vi "CAN_Init - EU.vi"(0 "设备类型":u32(ring)=4 items=["PCI5121"=1, "PCI9810"=2, "USBCAN1"=3, "USBCAN2"=4, "PCI9820"=5, "CAN232"=6, "PCI5110"=7, "CANLite(mini)"=8, "ISA9620"=9, "ISA5420"=10, "PC104CAN"=11, "CANET"=17, "DNP9810"=13, "USBCAN-E-U"=20, "USBCAN-2E-U"=21], 1 "设备索引":u32(ring) items=["0", "1", "2", "3", "4", "5", "6", "7", "8", "9", "10", "11", "12", "13", "14", "15", ""], 2 "波特率":T2(ring)=enum."250Kbps", 3 "CAN路数":u32(ring) items=["0", "1"], 4 "操作类型":enum16{"初始化CAN", "关闭CAN"}(ring), 5 "error in (no error)":errorcluster caption="错误输入（无错误）", 6 "滤波方式":u8(ring)=1 items=["Dual Filter", "Single Filter"], 7 "Accept Code":u32 format="%08x", 8 "IP":string, 9 "port":u32, 10 "工作方式":u8(ring) items=["Normal", "Listen Only"], 11 "Mask Code":u32=4294967295 format="%08x", 12 "PC端-协议类型":enum16{"TCP服务器Server", "TCP客户端Client"}(ring)) -> (14 "CAN 操作结果":bool=TRUE, 19 "error out":errorcluster caption="错误输出")   [LabVIEW 2013]
uses:
  data/ControlCAN.dll
panel:
  in  "VCI_INIT_CONFIG":T1={"AccCode"=0, "AccMask"=4294967295, "Reserved"=0, "Filter"=0, "Timing0"=191, "Timing1"=255, "Mode"=0}
  in  "DeviceType 5":u16(ring)=1 items=["PCI5121"=1, "PCI9810"=2, "USBCAN1"=3, "USBCAN2"=4, "PCI9820"=5, "CAN232"=6, "PCI5110"=7, "CANLite(mini)"=8, "ISA9620"=9, "ISA5420"=10, "PC104CAN"=11, "CANETE"=12, "DNP9810"=13]
  in  "CAN Channel 3":u16(ring) items=["0", "1"]
  in  "DeviceType 4":u16(ring)=1 items=["PCI5121"=1, "PCI9810"=2, "USBCAN1"=3, "USBCAN2"=4, "PCI9820"=5, "CAN232"=6, "PCI5110"=7, "CANLite(mini)"=8, "ISA9620"=9, "ISA5420"=10, "PC104CAN"=11, "CANETE"=12, "DNP9810"=13]
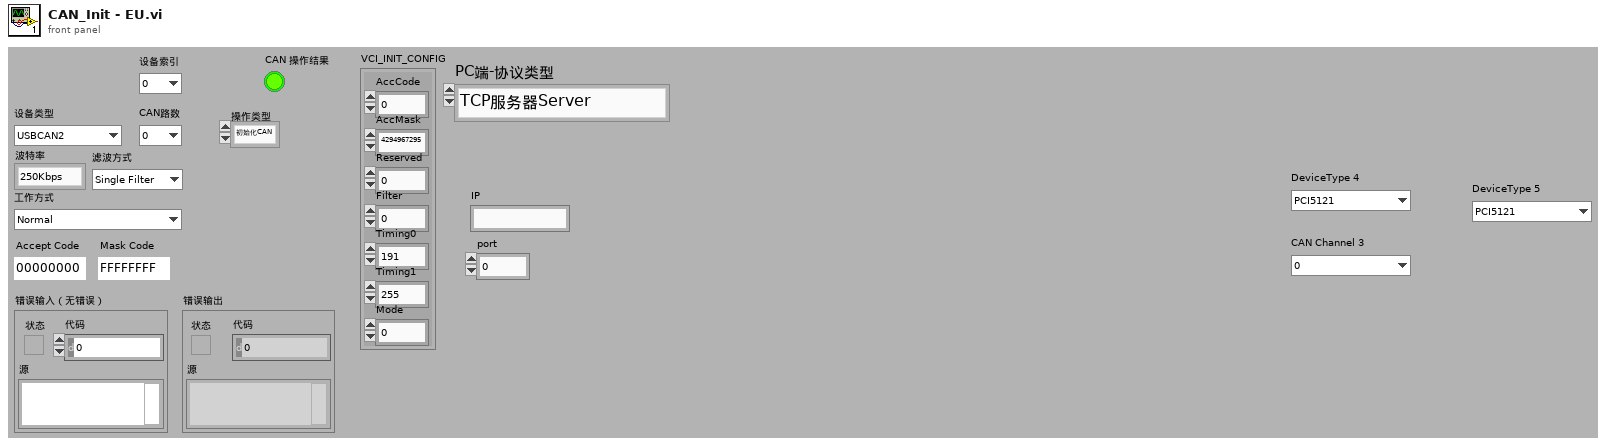
[diagram p1: front panel]
types:
  T1 = cluster{"AccCode":u32, "AccMask":u32, "Reserved":u32, "Filter":u8, "Timing0":u8, "Timing1":u8, "Mode":u8}
  T2 = enum16{"5Kbps", "10Kbps", "20Kbps", "40Kbps", "50Kbps", "80Kbps", "100Kbps", "125Kbps", "200Kbps", "250Kbps", "400Kbps", "500Kbps", "666Kbps", "800Kbps", "1000Kbps"}
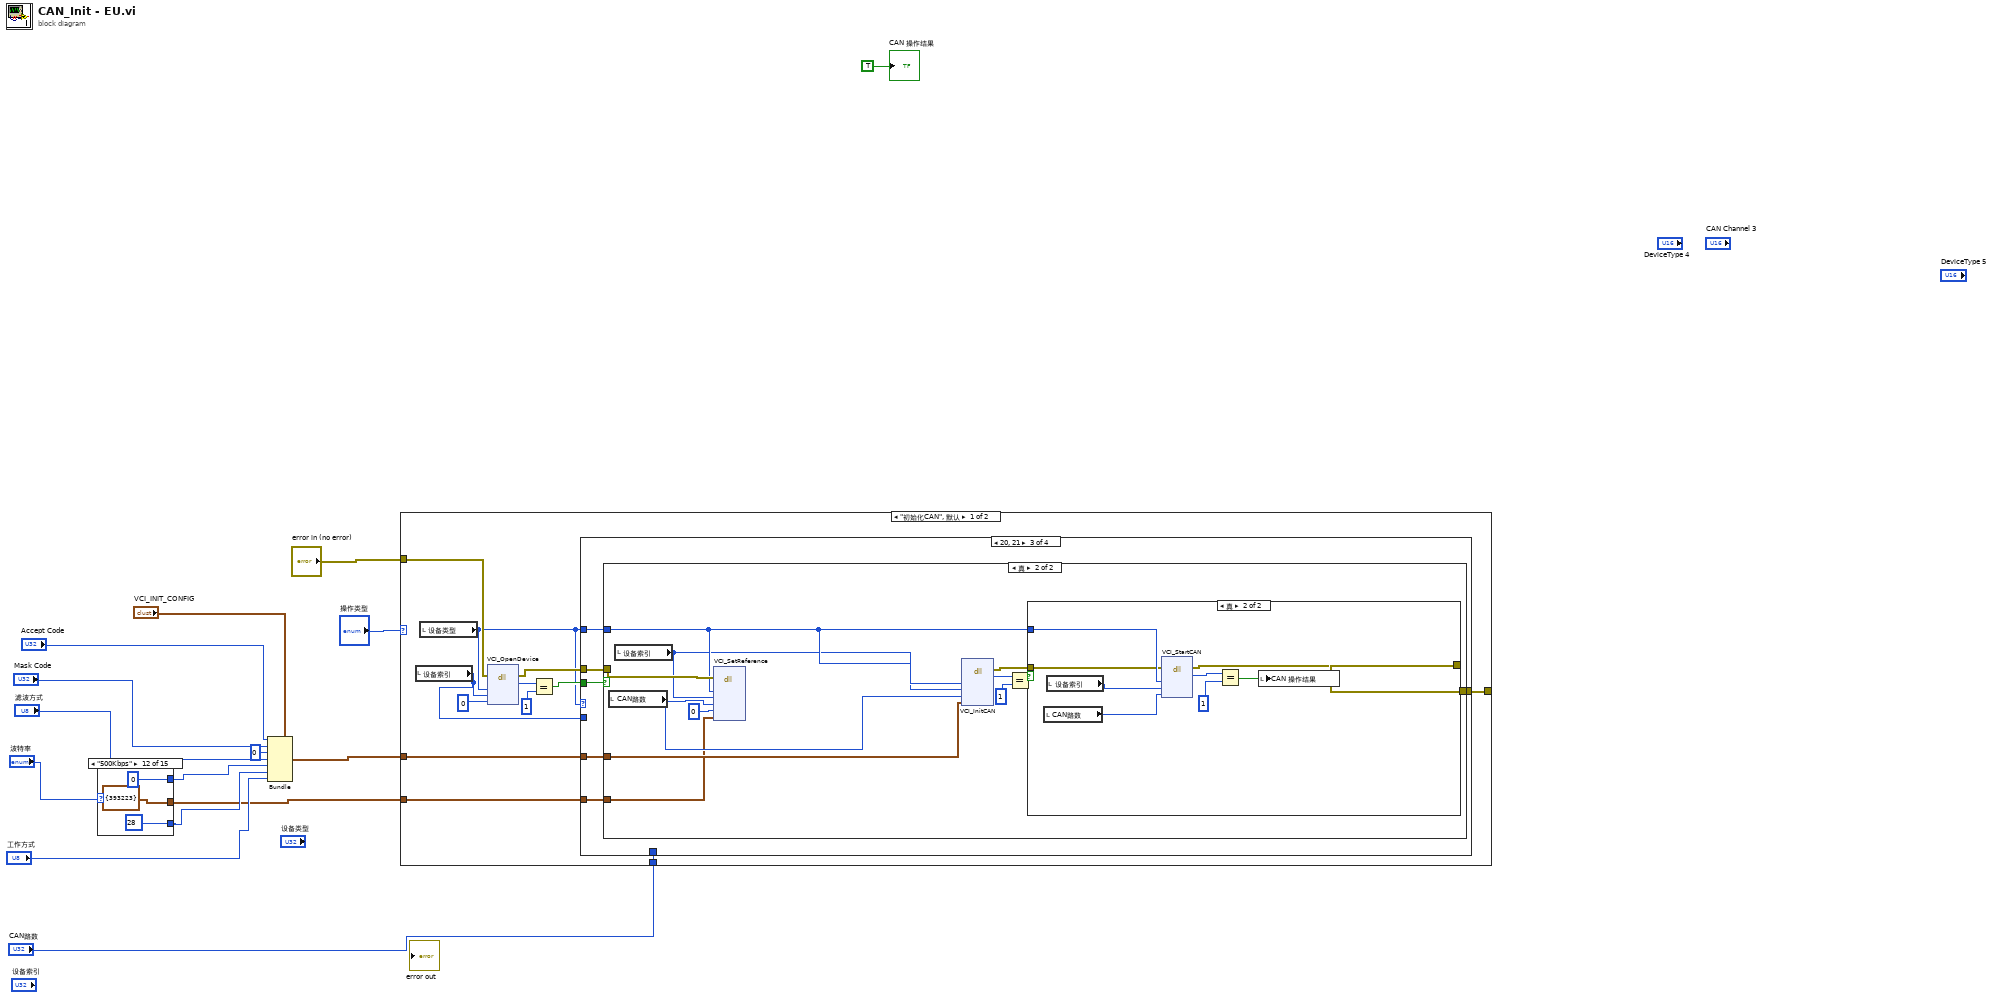
[diagram p0: block diagram]
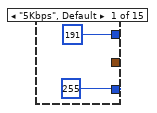
[diagram p2: hidden frame]
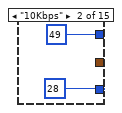
[diagram p3: hidden frame]
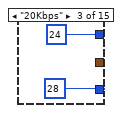
[diagram p4: hidden frame]
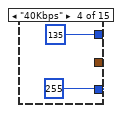
[diagram p5: hidden frame]
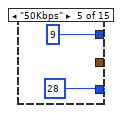
[diagram p6: hidden frame]
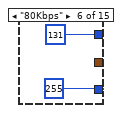
[diagram p7: hidden frame]
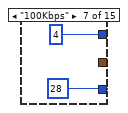
[diagram p8: hidden frame]
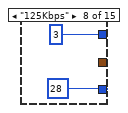
[diagram p9: hidden frame]
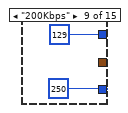
[diagram p10: hidden frame]
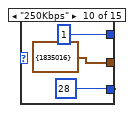
[diagram p11: hidden frame]
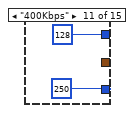
[diagram p12: hidden frame]
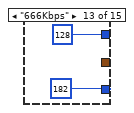
[diagram p13: hidden frame]
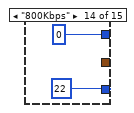
[diagram p14: hidden frame]
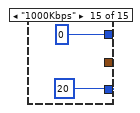
[diagram p15: hidden frame]
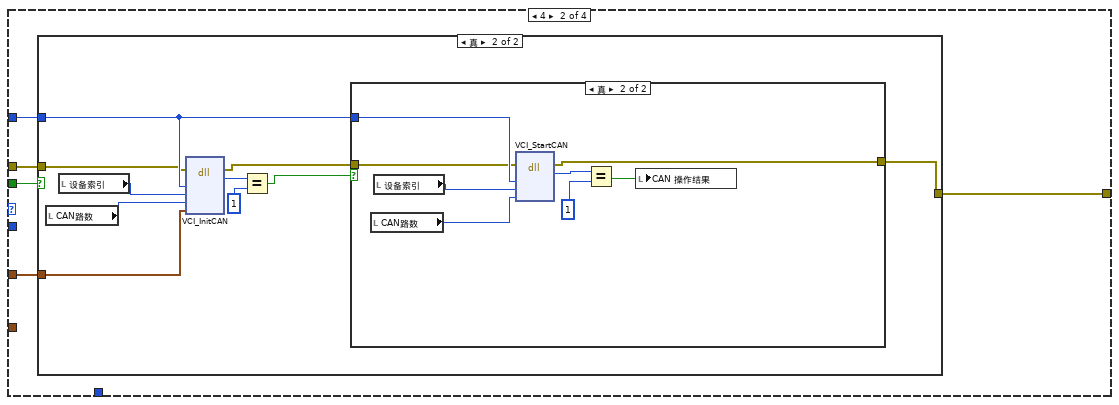
[diagram p17: hidden frame]
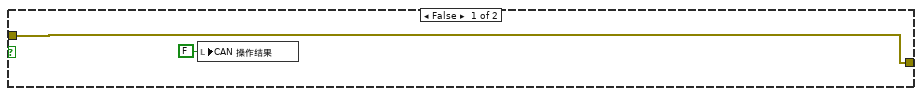
[diagram p18: hidden frame]
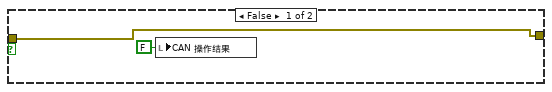
[diagram p19: hidden frame]
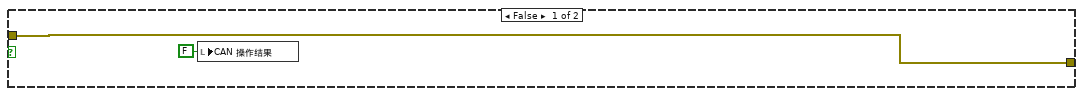
[diagram p20: hidden frame]
diagram:
  n1 = case shown="\"500Kbps\"" "波特率" {
    tunnel: [191 49 24 135 9 131 4 3 129 1 128 0 128 0 0] -> w14
    tunnel: [255 28 28 255 28 255 28 28 250 28 250 28 182 22 20] -> w13
    tunnel: [_ _ _ _ _ _ _ _ _ cluster{u32} {1835016} _ cluster{u32} {393223} _ _ _] -> w1
    frame "5Kbps", Default {
    }
    frame "10Kbps" {
    }
    frame "20Kbps" {
    }
    frame "40Kbps" {
    }
    frame "50Kbps" {
    }
    frame "80Kbps" {
    }
    frame "100Kbps" {
    }
    frame "125Kbps" {
    }
    frame "200Kbps" {
    }
    frame "250Kbps" {
    }
    frame "400Kbps" {
    }
    frame "500Kbps" {
    }
    frame "666Kbps" {
    }
    frame "800Kbps" {
    }
    frame "1000Kbps" {
    }
  }
  n2 = Bundle(cluster="VCI_INIT_CONFIG", "AccCode"="Accept Code", "AccMask"="Mask Code", "Reserved"=u32 0, "Filter"="滤波方式", "Timing0"=w14, "Timing1"=w13, "Mode"="工作方式") -> (w9:T1)
  n3 = case shown="\"初始化CAN\", 默认" "操作类型" {
    tunnel: w9 -> [w56 _]
    tunnel: "error in (no error)" -> [w55 w162]
    tunnel: [w53 w160] -> _
    tunnel: "CAN路数" -> [w50 _]
    tunnel: w1 -> [w48 _]
    frame "初始化CAN", Default {
      n4 = local read "设备索引"() -> (w51:u32)
      n5 = local read "设备类型"() -> (w49:u32)
      n6 = dll-call lib="PTH1Yabs FBluewave New Energy\t上位机BMS_Monitor - 91版 新源dataControlCAN.dll" fn="VCI_OpenDevice"(error in=w55, "DevType"=w49, "DevIndex"=w51, "Reserved"=0) -> (error out=w54:errorcluster, "返回类型"=w58:u32)  [unwired: 3 in, 3 out]
      n7 = Equal?(x=w58, y=u32 1) -> (x = y?=w52:bool)
      n8 = case shown="20, 21" w49 {
        tunnel: w52 -> [_ w65 w93 _]
        tunnel: w49 -> [_ w64 w92 w122]
        tunnel: w56 -> [_ w63 w91 _]
        tunnel: w54 -> [w60 w62 w90 w127]
        tunnel: [w60 w61 w89 w121] -> w53
        tunnel: w51 -> [_ _ _ w126]
        tunnel: w50 -> [_ _ _ w125]
        tunnel: w48 -> [_ _ w88 _]
        frame 0, Default {
        }
        frame 4 {
          n9 = case shown="真" w65 {
            tunnel: w64 -> [_ w72]
            tunnel: w63 -> [_ w71]
            tunnel: w62 -> [w66 w70]
            tunnel: [w66 w68] -> w61
            frame False {
              n10 = local write "CAN 操作结果"(FALSE ("初始化结果")) -> ()
            }
            frame True {
              n11 = local read "CAN路数"() -> (w74:u32)
              n12 = local read "设备索引"() -> (w75:u32)
              n13 = dll-call lib="PTH1Yabs FBluewave New Energy\t上位机BMS_Monitor - 91版 新源dataControlCAN.dll" fn="VCI_InitCAN"(error in=w70, "DeviceType"=w72, "DeviceInd"=w75, "CANInd"=w74, "pInitConfig"=w71) -> (error out=w69:errorcluster, "返回类型"=w76:u32)  [unwired: 3 in, 4 out]
              n14 = Equal?(x=w76, y=u32 1) -> (x = y?=w73:bool)
              n15 = case shown="真" w73 {
                tunnel: w72 -> [_ w85]
                tunnel: w69 -> [w78 w81]
                tunnel: [w78 w80] -> w68
                frame False {
                  n16 = local write "CAN 操作结果"(FALSE ("初始化结果")) -> ()
                }
                frame True {
                  n17 = local read "CAN路数"() -> (w83:u32)
                  n18 = local read "设备索引"() -> (w84:u32)
                  n19 = dll-call lib="PTH1Yabs FBluewave New Energy\t上位机BMS_Monitor - 91版 新源dataControlCAN.dll" fn="VCI_StartCAN"(error in=w81, "DeviceType"=w85, "DeviceInd"=w84, "CANInd"=w83) -> (error out=w80:errorcluster, "返回类型"=w86:u32)  [unwired: 2 in, 4 out]
                  n20 = Equal?(x=w86, y=u32 1) -> (x = y?=w82:bool)
                  n21 = local write "CAN 操作结果"(w82) -> ()
                }
              }
            }
          }
        }
        frame 20, 21 {
          n22 = case shown="真" w93 {
            tunnel: w92 -> [_ w99]
            tunnel: w91 -> [_ w104]
            tunnel: w90 -> [w94 w101]
            tunnel: [w94 w102] -> w89
            tunnel: w88 -> [_ w96]
            frame False {
              n23 = local write "CAN 操作结果"(FALSE ("初始化结果")) -> ()
            }
            frame True {
              n24 = local read "CAN路数"() -> (w97:u32)
              n25 = local read "设备索引"() -> (w98:u32)
              n26 = dll-call lib="PTH1Yabs FBluewave New Energy\t上位机BMS_Monitor - 91版 新源dataControlCAN.dll" fn="VCI_SetReference" label="VCI_SETREF"(error in=w101, "DeviceType"=w99, "DeviceInd"=w98, "CANInd"=w97, "RefType"=u32 0, "pData"=w96) -> ()  [unwired: 4 in, 6 out]
              n27 = dll-call lib="PTH1Yabs FBluewave New Energy\t上位机BMS_Monitor - 91版 新源dataControlCAN.dll" fn="VCI_InitCAN"("DeviceType"=w99, "DeviceInd"=w98, "CANInd"=w97, "pInitConfig"=w104) -> (error out=w103:errorcluster, "返回类型"=w106:u32)  [unwired: 4 in, 4 out]
              n28 = Equal?(x=w106, y=u32 1) -> (x = y?=w105:bool)
              n29 = case shown="真" w105 {
                tunnel: w99 -> [_ w115]
                tunnel: w103 -> [w108 w111]
                tunnel: [w108 w110] -> w102
                frame False {
                  n30 = local write "CAN 操作结果"(FALSE ("初始化结果")) -> ()
                }
                frame True {
                  n31 = local read "CAN路数"() -> (w113:u32)
                  n32 = local read "设备索引"() -> (w114:u32)
                  n33 = dll-call lib="PTH1Yabs FBluewave New Energy\t上位机BMS_Monitor - 91版 新源dataControlCAN.dll" fn="VCI_StartCAN"(error in=w111, "DeviceType"=w115, "DeviceInd"=w114, "CANInd"=w113) -> (error out=w110:errorcluster, "返回类型"=w116:u32)  [unwired: 2 in, 4 out]
                  n34 = Equal?(x=w116, y=u32 1) -> (x = y?=w112:bool)
                  n35 = local write "CAN 操作结果"(w112) -> ()
                }
              }
            }
          }
        }
        frame 17 {
          n36 = case shown="\"TCP客户端Client\", 默认" "PC端-协议类型" {
            tunnel: w127 -> [w138 w144]
            tunnel: w126 -> [w135 w141]
            tunnel: w125 -> [w134 w140]
            tunnel: [w132 w148] -> w124
            tunnel: [w131 w147] -> w123
            tunnel: w122 -> [w130 w142]
            tunnel: "IP" -> [w129 _]
            tunnel: "port" -> [w128 w146]
            frame "TCP客户端Client", Default {
              n37 = dll-call lib="PTH1Yabs FBluewave New Energy\t上位机BMS_Monitor - 91版 新源dataControlCAN.dll" fn="VCI_SetReference" label="VCI_SETREF"(error in=w138, "DeviceType"=w130, "DeviceInd"=w135, "CANInd"=w134, "RefType"=u32 0, "pData"=w129) -> (error out=w136:errorcluster)  [unwired: 4 in, 5 out]
              n38 = dll-call lib="PTH1Yabs FBluewave New Energy\t上位机BMS_Monitor - 91版 新源dataControlCAN.dll" fn="VCI_SetReference" label="VCI_SETREF"(error in=w136, "DeviceType"=w130, "DeviceInd"=w135, "CANInd"=w134, "RefType"=u32 1, "pData"=w128) -> (error out=w132:errorcluster, "返回类型"=w131:u32)  [unwired: 4 in, 4 out]
            }
            frame "TCP服务器Server" {
              n39 = dll-call lib="PTH1Yabs FBluewave New Energy\t上位机BMS_Monitor - 91版 新源dataControlCAN.dll" fn="VCI_SetReference" label="VCI_SETREF"(error in=w144, "DeviceType"=w142, "DeviceInd"=w141, "CANInd"=w140, "RefType"=u32 4, "pData"=u32 1) -> (error out=w143:errorcluster)  [unwired: 4 in, 5 out]
              n40 = dll-call lib="PTH1Yabs FBluewave New Energy\t上位机BMS_Monitor - 91版 新源dataControlCAN.dll" fn="VCI_SetReference" label="VCI_SETREF"(error in=w143, "DeviceType"=w142, "DeviceInd"=w141, "CANInd"=w140, "RefType"=u32 2, "pData"=w146) -> (error out=w148:errorcluster, "返回类型"=w147:u32)  [unwired: 4 in, 4 out]
            }
          }
          n41 = case shown="1" w123 {
            tunnel: w122 -> [_ w157]
            tunnel: w124 -> [w150 w153]
            tunnel: [w150 w152] -> w121
            frame 0, Default {
              n42 = local write "CAN 操作结果"(FALSE ("初始化结果")) -> ()
            }
            frame 1 {
              n43 = local read "CAN路数"() -> (w155:u32)
              n44 = local read "设备索引"() -> (w156:u32)
              n45 = dll-call lib="PTH1Yabs FBluewave New Energy\t上位机BMS_Monitor - 91版 新源dataControlCAN.dll" fn="VCI_StartCAN"(error in=w153, "DeviceType"=w157, "DeviceInd"=w156, "CANInd"=w155) -> (error out=w152:errorcluster, "返回类型"=w158:u32)  [unwired: 2 in, 4 out]
              n46 = Equal?(x=w158, y=u32 1) -> (x = y?=w154:bool)
              n47 = local write "CAN 操作结果"(w154) -> ()
            }
          }
        }
      }
    }
    frame "关闭CAN" {
      n48 = local read "CAN路数"() -> (w163:u32)
      n49 = local read "设备索引"() -> (w164:u32)
      n50 = local read "设备类型"() -> (w165:u32)
      n51 = dll-call lib="PTH1Yabs FBluewave New Energy\t上位机BMS_Monitor - 91版 新源dataControlCAN.dll" fn="VCI_ResetCAN"(error in=w162, "DeviceType"=w165, "DeviceInd"=w164, "CANInd"=w163) -> (error out=w161:errorcluster, "返回类型"=w167:u32)  [unwired: 2 in, 4 out]
      n52 = Equal?(x=w167, y=u32 1) -> (x = y?=w166:bool)
      n53 = case shown="真" w166 {
        tunnel: w161 -> [w169 w172]
        tunnel: [w169 w171] -> w160
        frame False {
          n54 = local write "CAN 操作结果"(FALSE ("CAN 操作结果")) -> ()
        }
        frame True {
          n55 = local read "设备类型"() -> (w175:u32)
          n56 = local read "设备索引"() -> (w174:u32)
          n57 = dll-call lib="PTH1Yabs FBluewave New Energy\t上位机BMS_Monitor - 91版 新源dataControlCAN.dll" fn="VCI_CloseDevice"(error in=w172, "DeviceType"=w175, "DeviceInd"=w174) -> (error out=w171:errorcluster, "返回类型"=w176:u32)  [unwired: 2 in, 3 out]
          n58 = Equal?(x=w176, y=u32 1) -> (x = y?=w173:bool)
          n59 = local write "CAN 操作结果"(w173) -> ()
        }
      }
    }
  }
  "CAN 操作结果" <- TRUE ("CAN 操作结果")
